vi "HMI.vi"(3 "Current Control settings":T1 {"Pump speed" format="%.2f"}) -> ()   [LabVIEW 2010]
uses:
  Stamp Controls.ctl
  switches.ctl
panel:
  in  "stop":bool
  # "what is this"
  # "rpm"
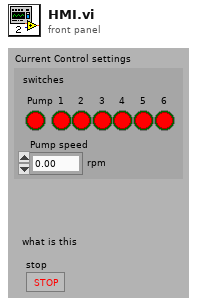
[diagram p1: front panel]
types:
  T1 = typedef "Stamp Controls.ctl" = cluster{"Pump speed":dbl, "switches":T2}
  T2 = typedef "switches.ctl" = cluster{"Pump":bool, "1":bool, "2":bool, "3":bool, "4":bool, "5":bool, "6":bool}
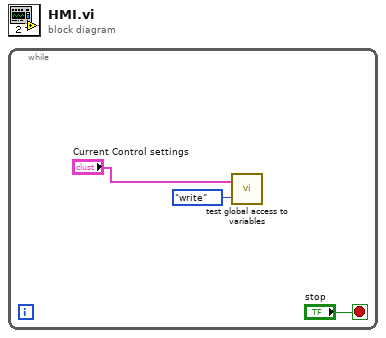
[diagram p0: block diagram]
diagram:
  n1 = while {
    stop <- "stop" stop-if-true
    n2 = call "test global access to variables.vi"("command"=enum16{"read", "write"}."write", "Current Control settings"="Current Control settings") -> ()  [unwired: 1 out]
  }
